vi "Get Name.vi"(8 "error in (no error)":errorcluster, 11 "Web FP In":refnum<class "Web Front Panel.lvclass">) -> (0 "error out":errorcluster, 2 "WFP Name":string, 3 "Web FP Out":refnum<class "Web Front Panel.lvclass">)   [LabVIEW 2017, in "Front Panel Publisher.lvlib" / "Web Front Panel.lvclass"]
uses:
  Web Front Panel.lvclass
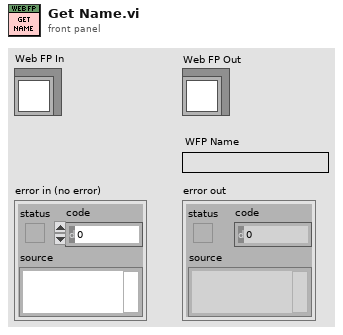
[diagram p1: front panel]
types:
  T1 = typedef "Front Panel Publisher.lvlib/Web Front Panel.lvclass/Object Attributes.ctl" = cluster{"VI Identifier":string, "VI Reference":refnum<vi>, "Controls":refnum<class "Object.lvclass">[], "Indicators":refnum<class "Object.lvclass">[], "Decorations":refnum<class "Object.lvclass">[], "VR With Previous Get":refnum<data-value>, "VR With Ring Images":refnum<data-value>}
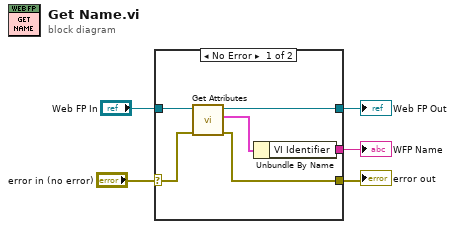
[diagram p0: block diagram]
diagram:
  n1 = case shown="No Error" "error in (no error)" {
    selector: "error in (no error)" -> [w11 w13]
    tunnel: [w9 w13] -> w4
    tunnel: [w7 w12] -> w2
    tunnel: "Web FP In" -> [w8 w12]
    tunnel: [w6 _] -> w1
    frame No Error {
      n2 = call "Get Attributes.vi"("error in (no error)"=w11, "Web FP In"=w8) -> ("error out"=w9:errorcluster, "Data"=w10:T1, "Web FP Out"=w7:refnum<class "Web Front Panel.lvclass">)  [unwired: 6 in, 1 out]
      n3 = Unbundle By Name(w10) -> ("VI Identifier"=w6:string)
    }
    frame Error {
    }
  }
  "error out" <- w4
  "Web FP Out" <- w2
  "WFP Name" <- w1
